vi "UnoLoopbackTesterv1.vi"() -> ()   [LabVIEW 2009]
uses:
  <vilib>/Instr/_visa.llb/VISA Configure Serial Port (Instr).vi
panel:
  in  "stop":bool
  in  "System":enum32{"Main", "Serial Terminal"}(tab)=enum."Serial Terminal"
  out "Outgoing Messages":string
  in  "Send":bool
  in  "Input":string
  in  "stop bits (10: 1 bit)":u16(ring)=10 items=["1.0"=10, "1.5"=15, "2.0"=20]
  in  "baud rate (9600)":u32=9600
  in  "parity (0:none)":enum16{"None", "Odd", "Even", "Mark", "Space"}(ring)
  in  "data bits (8)":u16=8 min=5 max=8 step=1
  in  "VISA resource name":refnum<visa-resource-name>
  out "Incoming Messages":string
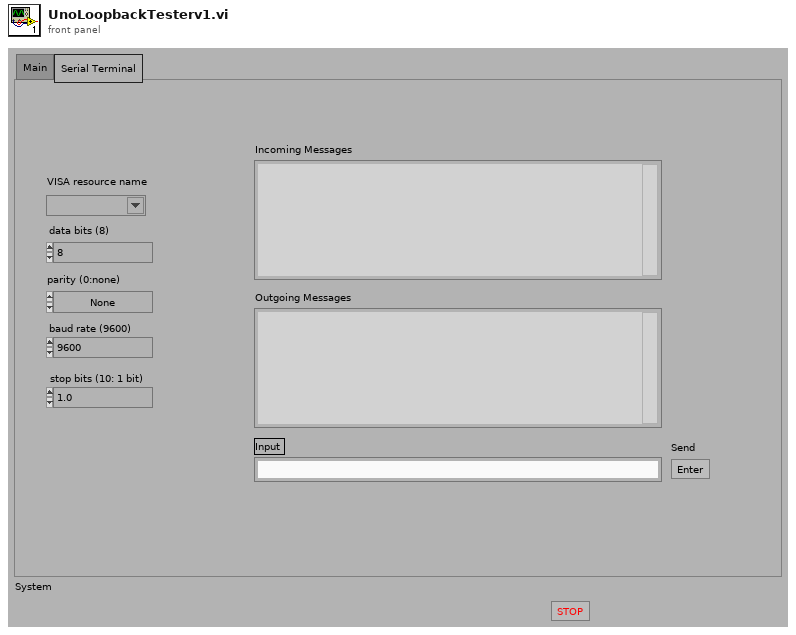
[diagram p1: front panel]
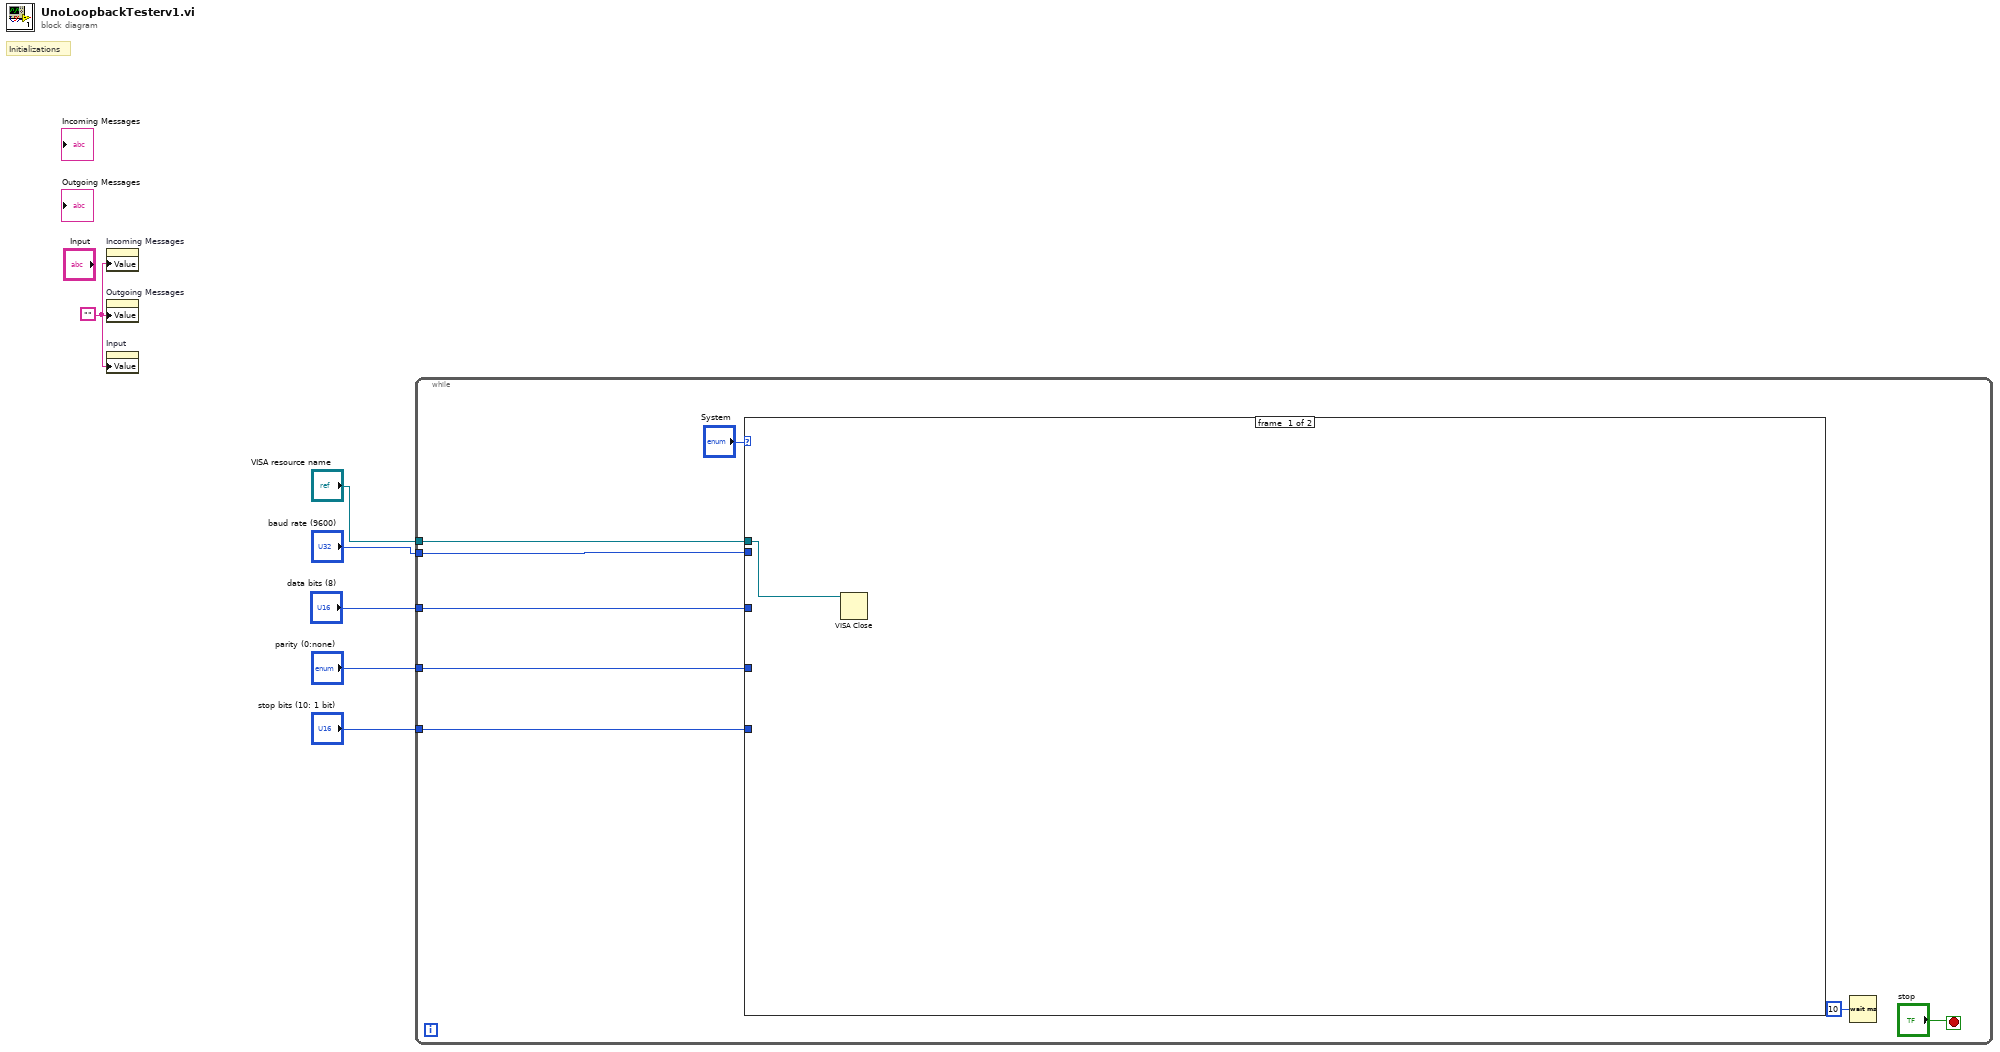
[diagram p0: block diagram]
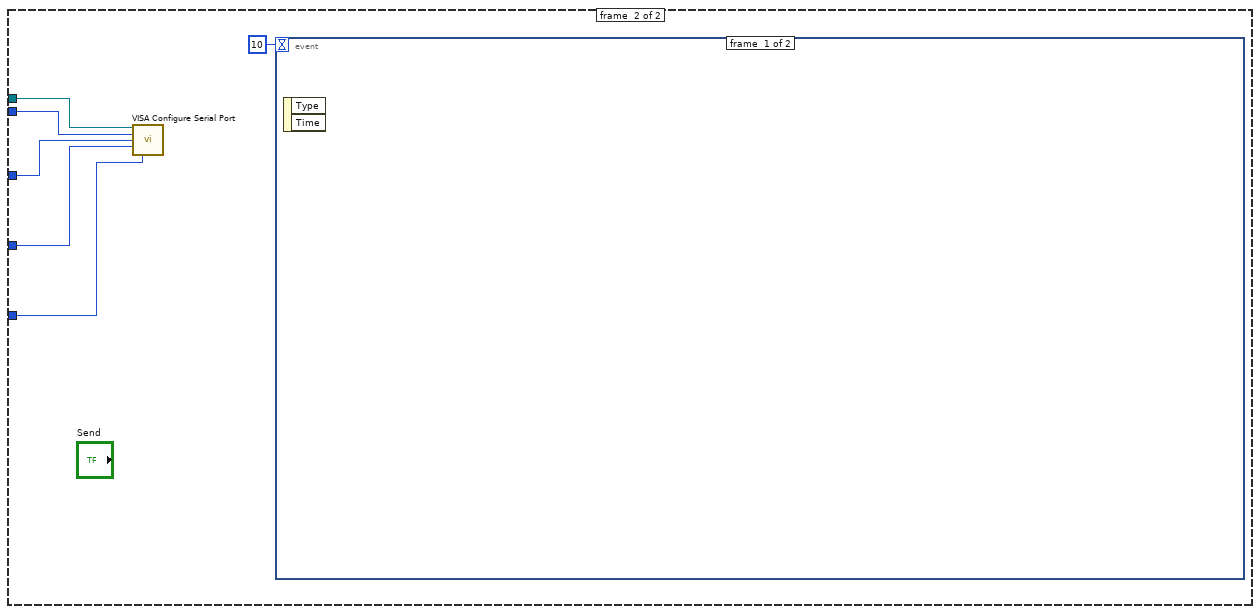
[diagram p2: hidden frame]
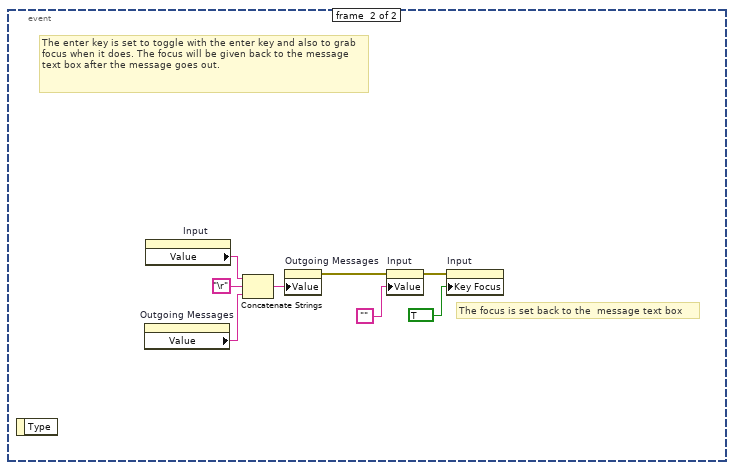
[diagram p3: hidden frame]
diagram:
  w1 = ""
  # "Initializations"
  n1 = property on="Incoming Messages" class="Str"("Value"=w1) -> ()  [unwired: 2 in, 2 out]
  n2 = property on="Outgoing Messages" class="Str"("Value"=w1) -> ()  [unwired: 2 in, 2 out]
  n3 = property on="Input" class="Str"("Value"=w1) -> ()  [unwired: 2 in, 2 out]
  n4 = while {
    tunnel: "VISA resource name" -> [w11]
    tunnel: "baud rate (9600)" -> [w10]
    tunnel: "data bits (8)" -> [w9]
    tunnel: "parity (0:none)" -> [w8]
    tunnel: "stop bits (10: 1 bit)" -> [w7]
    stop <- "stop" stop-if-true
    n5 = case shown="\"Serial Terminal\"" "System" {
      tunnel: w11 -> [w15 w19]
      tunnel: w10 -> [_ w21]
      tunnel: w9 -> [_ w20]
      tunnel: w8 -> [_ w18]
      tunnel: w7 -> [_ w17]
      frame #0 {
        n6 = VISA Close(VISA resource name=w15) -> ()  [unwired: 1 in, 1 out]
      }
      frame #1 {
        n7 = call-poly "VISA Configure Serial Port"("VISA resource name"=w19, "baud rate (9600)"=w21, "data bits (8)"=w20, "parity (0:none)"=w18, "stop bits (10: 1 bit)"=w17) -> ()  [unwired: 9 in, 2 out]
        n8 = event shown="[1] \"Send\": Value Change" {
          selector: _ -> [_ _]
          dyn-events: _ -> [_ _]
          timeout: 10 -> [_ _]
          event #0 {
            n9 = event-data() -> ()  [unwired: 1 in, 2 out]
          }
          event #1 {
            # "The enter key is set to toggle with the enter key and also to grab focus when it does. The focus will be given back to the message text box after the message goes out."
            # "The focus is set back to the  message text box"
            n10 = event-data() -> ()  [unwired: 1 in, 1 out]
            n11 = property on="Outgoing Messages" class="Str"() -> ("Value"=w24:string)  [unwired: 2 in, 2 out]
            n12 = property on="Input" class="Str"() -> ("Value"=w26:string)  [unwired: 2 in, 2 out]
            n13 = Concatenate Strings(w26, "\r", w24) -> (w28:string)
            n14 = property on="Outgoing Messages" class="Str"("Value"=w28) -> (error out=w29:errorcluster)  [unwired: 2 in, 1 out]
            n15 = property on="Input" class="Str"(error in=w29, "Value"="") -> (error out=w22:errorcluster)  [unwired: 1 in, 1 out]
            n16 = property on="Input" class="Str"(error in=w22, "Key Focus"=TRUE) -> ()  [unwired: 1 in, 2 out]
          }
        }
      }
    }
    n17 = Wait (ms)(milliseconds to wait=u32 10) -> ()  [unwired: 1 out]
  }
